vi "ic初始化.vi"(10 "路径":path, 11 "自动化引用句柄输入":refnum<k7>) -> (2 "自动化引用句柄输入 2":refnum<k7>)   [LabVIEW 2014]
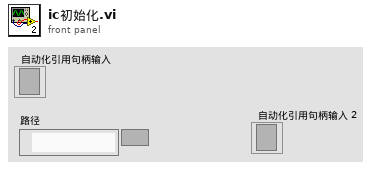
[diagram p1: front panel]
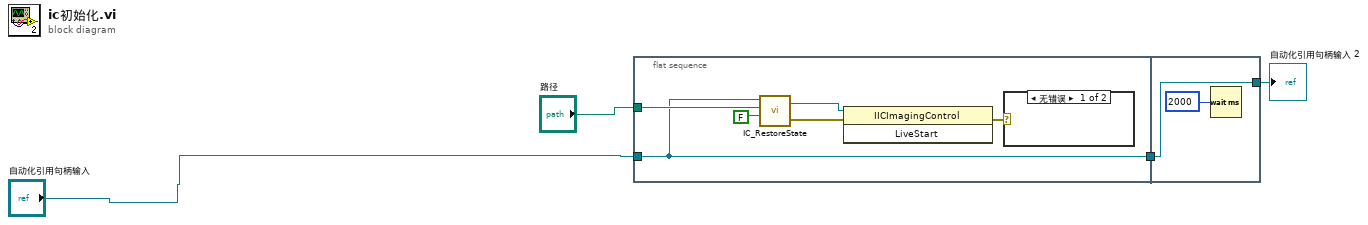
[diagram p0: block diagram]
diagram:
  n1 = flat-sequence {
    tunnel: "路径" -> [w7]
    tunnel: "自动化引用句柄输入" -> [w5]
    tunnel: [w5] -> w4
    tunnel: [w11] -> w1
    tunnel: w4 -> [w11]
    frame #0 {
      n2 = call "IC_RestoreState.vi"("Color"=FALSE, "File Path"=w7, "ICImagingControl"=w5) -> ("Error Out"=w8:errorcluster, "ICImagingControl Out"=w9:refnum<k7>)  [unwired: 1 in]
      n3 = invoke class="IICImagingControl" method="LiveStart"(reference=w9, error in=w8) -> (error out=w6:errorcluster)  [unwired: 1 in, 2 out]
      n4 = case shown="无错误" w6 {
        frame No Error {
        }
        frame Error {
        }
      }
    }
    frame #1 {
      n5 = Wait (ms)(milliseconds to wait=u32 2000 ("等待时间（毫秒）")) -> ()  [unwired: 1 out]
    }
  }
  "自动化引用句柄输入 2" <- w1
